vi "pulse_test.vi"() -> ()   [LabVIEW 2012]
uses:
  <vilib>/DAQmx/write.llb/DAQmx Write (Digital Bool 1Line 1Point).vi
  <vilib>/DAQmx/create/channels.llb/DAQmx Create Channel (DO-Digital Output).vi
  <vilib>/DAQmx/miscellaneous.llb/DAQmx Fill In Error Info.vi
  MagiQmw3.lvclass
panel:
  out "Numeric":i32
  in  "stop":bool
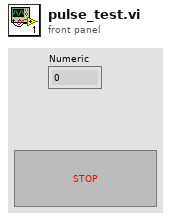
[diagram p1: front panel]
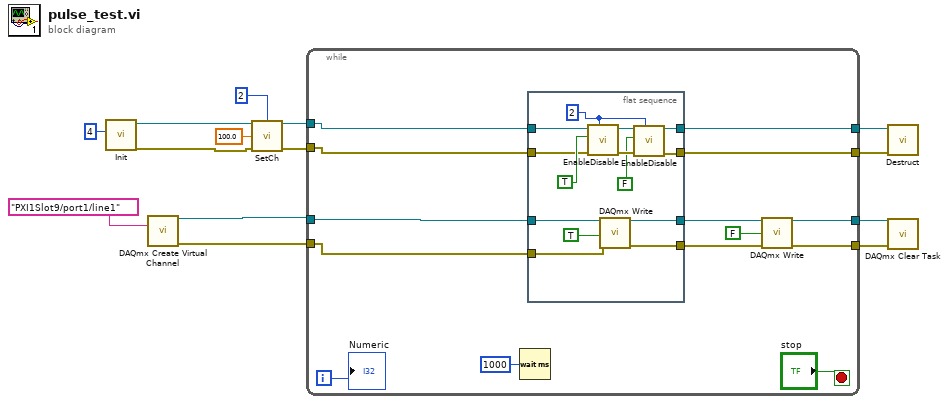
[diagram p0: block diagram]
diagram:
  n1 = call "Init.vi"("Slot"=u16 4) -> ("error out"=w4:errorcluster, "MagiQmw3 out"=w3:refnum<class "MagiQmw3.lvclass">)  [unwired: 9 in]
  n2 = call-poly <vilib>:"DAQmx Create Virtual Channel.vi"("lines"=tag "PXI1Slot9/port1/line1") -> ("task out"=w2:refnum<k21>, "error out"=w1:errorcluster)  [unwired: 13 in]
  n3 = call "SetCh.vi"("MagiQmw3 in"=w3, "ch"=2, "freq"=100.0, "error in (no error)"=w4) -> ("MagiQmw3 out"=w6:refnum<class "MagiQmw3.lvclass">, "error out"=w5:errorcluster)  [unwired: 10 in]
  n4 = while {
    tunnel: w5 -> [w19]
    tunnel: w6 -> [w20]
    tunnel: [w28] -> w14
    tunnel: [w27] -> w13
    tunnel: w2 -> [w18]
    tunnel: [w25] -> w11
    tunnel: [w24] -> w10
    tunnel: w1 -> [w15]
    i -> [w22]
    stop <- "stop" stop-if-true
    n5 = Wait (ms)(milliseconds to wait=u32 1000) -> ()  [unwired: 1 out]
    n6 = flat-sequence {
      tunnel: [w38] -> w28
      tunnel: [w37] -> w27
      tunnel: w20 -> [w35]
      tunnel: w19 -> [w34]
      tunnel: w18 -> [w32]
      tunnel: [w31] -> w17
      tunnel: [w30] -> w16
      tunnel: w15 -> [w29]
      frame #0 {
        w39 = 2 ("ch")
        n7 = call "EnableDisable.vi"("ch"=w39, "error in (no error)"=w34, "Enable"=TRUE, "MagiQmw3 in"=w35) -> ("error out"=w40:errorcluster, "MagiQmw3 out"=w41:refnum<class "MagiQmw3.lvclass">)  [unwired: 6 in]
        n8 = call-poly <vilib>:"DAQmx Write.vi"("task/channels in"=w32, "data"=TRUE, "error in"=w29) -> ("task out"=w30:refnum<k21>, "error out"=w31:errorcluster)  [unwired: 10 in, 1 out]
        n9 = call "EnableDisable.vi"("ch"=w39, "error in (no error)"=w40, "Enable"=FALSE, "MagiQmw3 in"=w41) -> ("error out"=w37:errorcluster, "MagiQmw3 out"=w38:refnum<class "MagiQmw3.lvclass">)  [unwired: 6 in]
      }
    }
    n10 = call-poly <vilib>:"DAQmx Write.vi"("task/channels in"=w16, "data"=FALSE, "error in"=w17) -> ("task out"=w24:refnum<k21>, "error out"=w25:errorcluster)  [unwired: 10 in, 1 out]
    "Numeric" <- w22
  }
  n11 = call "Destruct.vi"("error in (no error)"=w13, "MagiQmw3 in"=w14) -> ()  [unwired: 9 in, 1 out]
  n12 = call <vilib>:"DAQmx Clear Task.vi"("task in"=w10, "error in"=w11) -> ()  [unwired: 13 in, 1 out]
